vi "PathPlanner_TrajectoryState25_New.vi"(0 "PathPlannerConstraints":T8={"MaxVelocityMps;"=0.0, "MaxAccelerationMpsSq;"=0.0, "MaxAngularVelRadPsEc;"=0.0, "MaxAngularAccRadPSecSq"=0.0, "Exists"=FALSE, "Unlimited"=FALSE, "NominalVoltageVolts"=12.0}, 1 "WaypointRelPos":dbl, 3 "TimeSeconds":dbl, 4 "ModuleStates":T1[](array[typedef]) {"SWERVE_DRIVE_MODULE_STATE"."Angle"."SIN" format="%13.4f"; "SWERVE_DRIVE_MODULE_STATE"."Angle"."COS" format="%13.4f"; "SWERVE_DRIVE_MODULE_STATE"."Angle"."VALUE" format="%13.4f"; "FieldAngle"."SIN" format="%13.4f"; "FieldAngle"."COS" format="%13.4f"; "FieldAngle"."VALUE" format="%13.4f"; "FieldPos"."Y" format="%14.3f"; "FieldPos"."X" format="%14.3f"}, 5 "FieldSpeeds":T7 {"vOmega" format="%10.3f"; "vY" format="%10.3f"; "vX" format="%10.3f"}, 6 "DeltaRot":T3={"VALUE"=0.0, "COS"=1.0, "SIN"=0.0} {"SIN" format="%13.4f"; "COS" format="%13.4f"; "VALUE" format="%13.4f"}, 7 "pose":T6={"TRANSLATION"={"X"=0.0, "Y"=0.0}, "ROTATION"={"VALUE"=0.0, "COS"=1.0, "SIN"=0.0}} {"ROTATION"."SIN" format="%13.4f"; "ROTATION"."COS" format="%13.4f"; "ROTATION"."VALUE" format="%13.4f"; "TRANSLATION"."Y" format="%14.3f"; "TRANSLATION"."X" format="%14.3f"}, 8 "DeltaPos":dbl, 9 "Feedforwards":T5, 10 "Heading":T3={"VALUE"=0.0, "COS"=1.0, "SIN"=0.0} {"SIN" format="%13.4f"; "COS" format="%13.4f"; "VALUE" format="%13.4f"}, 11 "LinearVelocity":dbl) -> (2 "PathPlannerState":T9={"TimeSeconds"=0.0, "LinearVelocity"=0.0, "Heading"={"VALUE"=0.0, "COS"=1.0, "SIN"=0.0}, "Constraints"={"MaxVelocityMps;"=0.0, "MaxAccelerationMpsSq;"=0.0, "MaxAngularVelRadPsEc;"=0.0, "MaxAngularAccRadPSecSq"=0.0, "Exists"=FALSE, "Unlimited"=FALSE, "NominalVoltageVolts"=12.0}, "DeltaPos"=0.0, "FieldSpeeds"={"vX"=0.0, "vY"=0.0, "vOmega"=0.0}, "pose"={"TRANSLATION"={"X"=0.0, "Y"=0.0}, "ROTATION"={"VALUE"=0.0, "COS"=1.0, "SIN"=0.0}}, "DeltaRot"={"VALUE"=0.0, "COS"=1.0, "SIN"=0.0}, "ModuleStates"=[], "WaypointRelPos"=0.0, "Feedforwards"={"accelerationsMPSSq"=[], "linearForcesNewtons"=[], "torqueCurrentsAmps"=[], "robotRelativeForcesXNewtons"=[], "robotRelativeForcesYNewtons"=[]}} {"ModuleStates"."SWERVE_DRIVE_MODULE_STATE"."Angle"."SIN" format="%13.4f"; "ModuleStates"."SWERVE_DRIVE_MODULE_STATE"."Angle"."COS" format="%13.4f"; "ModuleStates"."SWERVE_DRIVE_MODULE_STATE"."Angle"."VALUE" format="%13.4f"; "ModuleStates"."FieldAngle"."SIN" format="%13.4f"; "ModuleStates"."FieldAngle"."COS" format="%13.4f"; "ModuleStates"."FieldAngle"."VALUE" format="%13.4f"; "ModuleStates"."FieldPos"."Y" format="%14.3f"; "ModuleStates"."FieldPos"."X" format="%14.3f"; "DeltaRot"."SIN" format="%13.4f"; "DeltaRot"."COS" format="%13.4f"; "DeltaRot"."VALUE" format="%13.4f"; "pose"."ROTATION"."SIN" format="%13.4f"; "pose"."ROTATION"."COS" format="%13.4f"; "pose"."ROTATION"."VALUE" format="%13.4f"; "pose"."TRANSLATION"."Y" format="%14.3f"; "pose"."TRANSLATION"."X" format="%14.3f"; "FieldSpeeds"."vOmega" format="%10.3f"; "FieldSpeeds"."vY" format="%10.3f"; "FieldSpeeds"."vX" format="%10.3f"; "Heading"."SIN" format="%13.4f"; "Heading"."COS" format="%13.4f"; "Heading"."VALUE" format="%13.4f"})   [LabVIEW 2019, in "PathPlanner24.lvlib"]
doc: "Create a trajectory state\n\nInputs:\n -- timeSeconds - double - The time at this state in seconds ( default = 0; )\n -- velocityMps - double - The velocity at this state in m/s ( default = 0 )\n -- accelerationMpsSq - double - The acceleration at this state in m/s^2 ( default = 0 )\n -- headingAngularVelocityRps - double - The time at this state in seconds ( default = 0 )\n -- positionMeters - translation2d - The position at this state in meters ( default = 0,0 )\n -- heading - rotation2d - The heading (direction of travel) at this state ( default = 0 )\n -- targetHolonomicRotation - rotation2d - The target holonomic rotation at this state ( default = 0 )\n -- curvatureRadPerMeter - double - The curvature at this state in rad/m ( default = 0 )\n -- constraints -- cluster -- constraints to apply at this state (default - none )\n - WaypointRelPos - double - The waypoint relative pos for this state.\n\n\nOutputs\n - PathPlannerTrajectoryState -- cluster -- Newly created state"
uses:
  PathPlanner24.lvlib
  TypeDef/PathPlannerTrajectoryState25.ctl
  <vilib>/Rock Robotics/WPI/ThirdParty/JAS_Junk/TrajLib/TypeDef/ROTATION2D.ctl
  TypeDef/PathPlannerPathConstraints.ctl
  <vilib>/Rock Robotics/WPI/ThirdParty/JAS_Junk/TrajLib/TypeDef/CHASSIS_SPEEDS.ctl
  <vilib>/Rock Robotics/WPI/ThirdParty/JAS_Junk/TrajLib/TypeDef/POSE2D.ctl
  <vilib>/Rock Robotics/WPI/ThirdParty/JAS_Junk/TrajLib/TypeDef/TRANSLATION2D.ctl
  TypeDef/PathPlannerSwerveModTrajState.ctl
  <vilib>/Rock Robotics/WPI/ThirdParty/JAS_Junk/TrajLib/TypeDef/SWERVE_DRIVE_MODULE_STATE.ctl
  TypeDef/PathPlannerDriveFeedFwds.ctl
  <vilib>/Rock Robotics/WPI/ThirdParty/JAS_Junk/TrajLib/Trajectory_Library.lvlib
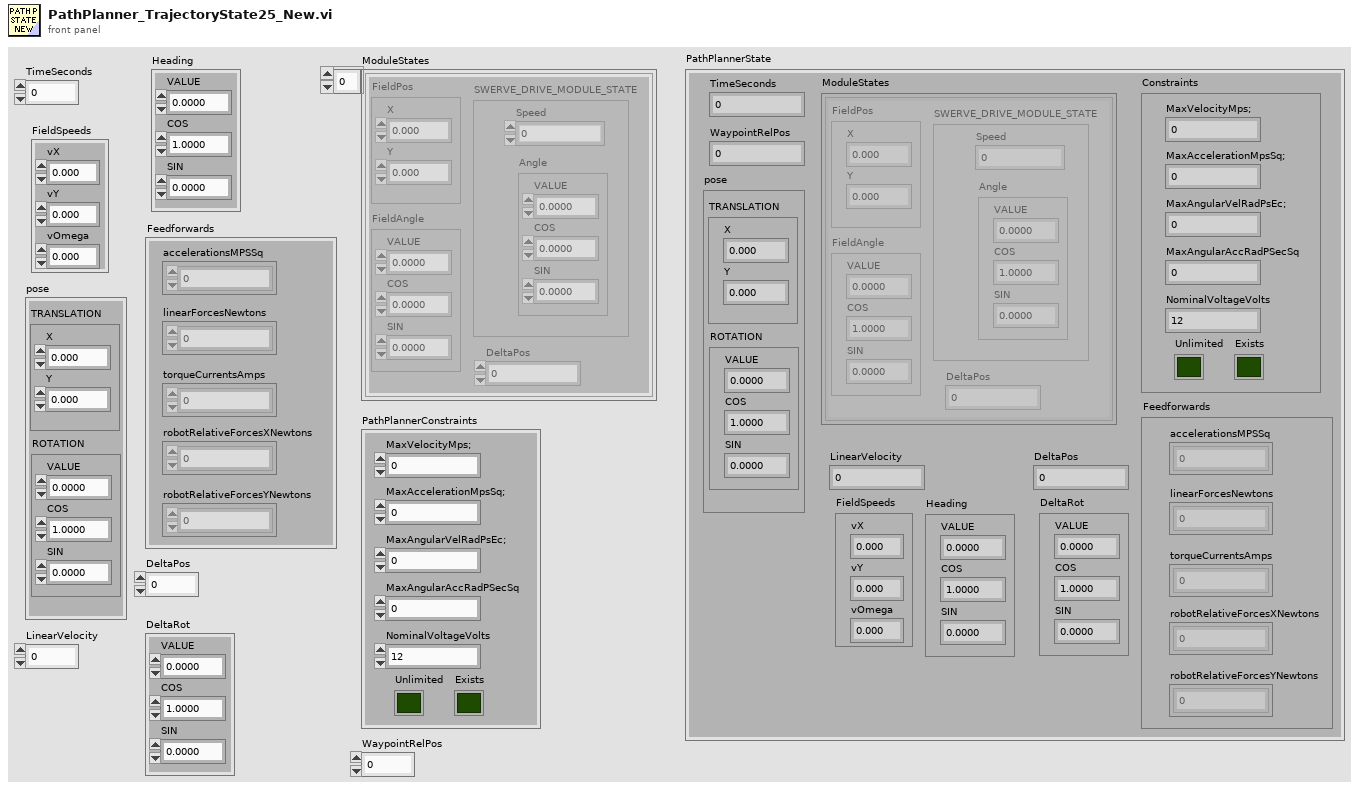
[diagram p1: front panel]
types:
  T1 = typedef "PathPlanner24.lvlib/PathPlannerSwerveModTrajState.ctl" = cluster{"FieldPos":T2, "FieldAngle":T3, "DeltaPos":dbl, "SWERVE_DRIVE_MODULE_STATE":T4}
  T2 = typedef "Trajectory_Library.lvlib/TRANSLATION2D.ctl" = cluster{"X":dbl, "Y":dbl}
  T3 = typedef "Trajectory_Library.lvlib/ROTATION2D.ctl" = cluster{"VALUE":dbl, "COS":dbl, "SIN":dbl}
  T4 = typedef "Trajectory_Library.lvlib/SWERVE_DRIVE_MODULE_STATE.ctl" = cluster{"Speed":dbl, "Angle":T3}
  T5 = typedef "PathPlanner24.lvlib/PathPlannerDriveFeedFwds.ctl" = cluster{"accelerationsMPSSq":dbl[], "linearForcesNewtons":dbl[], "torqueCurrentsAmps":dbl[], "robotRelativeForcesXNewtons":dbl[], "robotRelativeForcesYNewtons":dbl[]}
  T6 = typedef "Trajectory_Library.lvlib/POSE2D.ctl" = cluster{"TRANSLATION":T2, "ROTATION":T3}
  T7 = typedef "Trajectory_Library.lvlib/CHASSIS_SPEEDS.ctl" = cluster{"vX":dbl, "vY":dbl, "vOmega":dbl}
  T8 = typedef "PathPlanner24.lvlib/PathPlannerPathConstraints.ctl" = cluster{"MaxVelocityMps;":dbl, "MaxAccelerationMpsSq;":dbl, "MaxAngularVelRadPsEc;":dbl, "MaxAngularAccRadPSecSq":dbl, "Exists":bool, "Unlimited":bool, "NominalVoltageVolts":dbl}
  T9 = typedef "PathPlanner24.lvlib/PathPlannerTrajectoryState25.ctl" = cluster{"TimeSeconds":dbl, "LinearVelocity":dbl, "Heading":T3, "Constraints":T8, "DeltaPos":dbl, "FieldSpeeds":T7, "pose":T6, "DeltaRot":T3, "ModuleStates":T1[], "WaypointRelPos":dbl, "Feedforwards":T5}
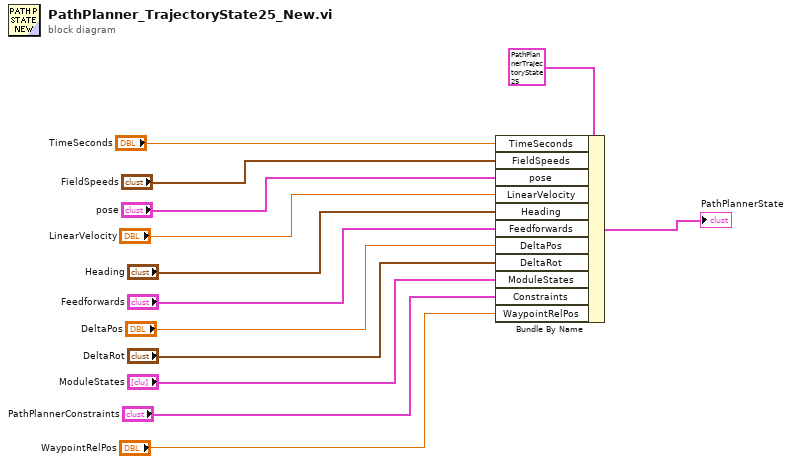
[diagram p0: block diagram]
diagram:
  n1 = Bundle By Name(cluster=T9 {"TimeSeconds"=0.0, "LinearVelocity"=0.0, "Heading"={"VALUE"=0.0, "COS"=1.0, "SIN"=0.0}, "Constraints"={"MaxVelocityMps;"=0.0, "MaxAccelerationMpsSq;"=0.0, "MaxAngularVelRadPsEc;"=0.0, "MaxAngularAccRadPSecSq"=0.0, "Exists"=FALSE, "Unlimited"=FALSE, "NominalVoltageVolts"=12.0}, "DeltaPos"=0.0, "FieldSpeeds"={"vX"=0.0, "vY"=0.0, "vOmega"=0.0}, "pose"={"TRANSLATION"={"X"=0.0, "Y"=0.0}, "ROTATION"={"VALUE"=0.0, "COS"=1.0, "SIN"=0.0}}, "DeltaRot"={"VALUE"=0.0, "COS"=1.0, "SIN"=0.0}, "ModuleStates"=[], "WaypointRelPos"=0.0, "Feedforwards"={"accelerationsMPSSq"=[], "linearForcesNewtons"=[], "torqueCurrentsAmps"=[], "robotRelativeForcesXNewtons"=[], "robotRelativeForcesYNewtons"=[]}} ("PathPlannerState"), "TimeSeconds"="TimeSeconds", "FieldSpeeds"="FieldSpeeds", "pose"="pose", "LinearVelocity"="LinearVelocity", "Heading"="Heading", "Feedforwards"="Feedforwards", "DeltaPos"="DeltaPos", "DeltaRot"="DeltaRot", "ModuleStates"="ModuleStates", "Constraints"="PathPlannerConstraints", "WaypointRelPos"="WaypointRelPos") -> (→"PathPlannerState":T9)
